vi "Get TableVariable Name List.vi"(8 "error in (no error)":errorcluster, 11 "DataTable":refnum<k7>) -> (0 "error out":errorcluster, 2 "TableVariable name list":string[](array[string]), 3 "DataTable out":refnum<k7>)   [LabVIEW 2019, in "JMP Automation.lvlib"]
doc: "retreive the name list of the TableVariable from a DataTable. The DataTable will be \"activated\" (put on the front) during the opperation\n\nDataTable: valide DataTable application handle"
uses:
  JMP Automation.lvlib
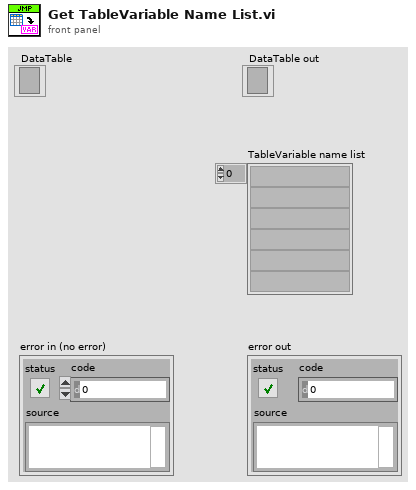
[diagram p1: front panel]
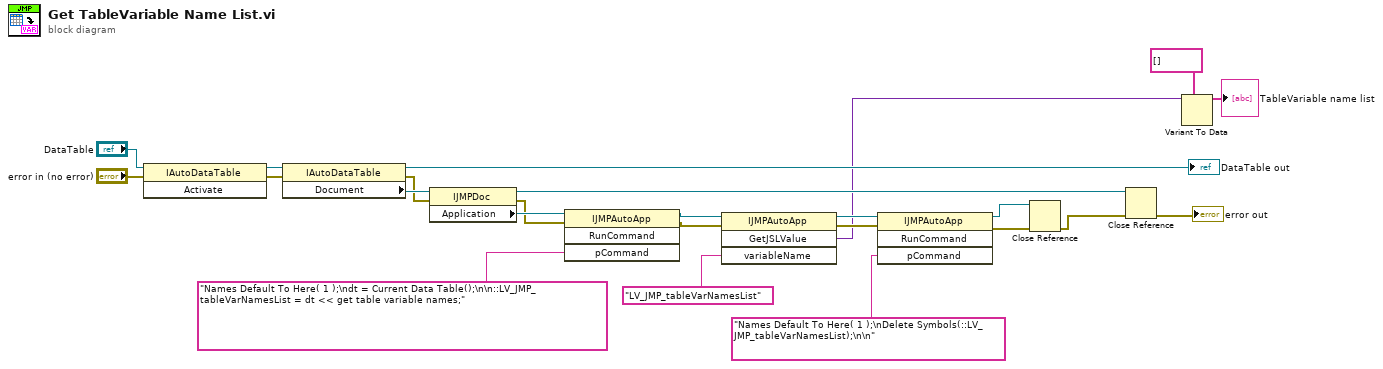
[diagram p0: block diagram]
diagram:
  n1 = invoke class="IAutoDataTable" method="Activate"(reference="DataTable", error in="error in (no error)") -> (reference out=w21:refnum<k7>, error out=w23:errorcluster)  [unwired: 1 in, 1 out]
  n2 = property class="IAutoDataTable"(reference=w21, error in=w23) -> (reference out=→"DataTable out":refnum<k7>, error out=w18:errorcluster, "Document"=w20:refnum<k7>)
  n3 = property class="IJMPDoc"(reference=w20, error in=w18) -> (reference out=w5:refnum<k7>, error out=w17:errorcluster, "Application"=w19:refnum<k7>)
  n4 = invoke class="IJMPAutoApp" method="RunCommand"(reference=w19, error in=w17, "pCommand"="Names Default To Here( 1 );\ndt = Current Data Table();\n\n::LV_JMP_tableVarNamesList = dt << get table variable names;") -> (reference out=w11:refnum<k7>, error out=w10:errorcluster)  [unwired: 1 in, 2 out]
  n5 = invoke class="IJMPAutoApp" method="GetJSLValue"(reference=w11, error in=w10, "variableName"="LV_JMP_tableVarNamesList") -> (reference out=w9:refnum<k7>, error out=w8:errorcluster, "GetJSLValue"=w1:variant)  [unwired: 1 in, 1 out]
  n6 = invoke class="IJMPAutoApp" method="RunCommand"(reference=w9, error in=w8, "pCommand"="Names Default To Here( 1 );\nDelete Symbols(::LV_JMP_tableVarNamesList);\n\n") -> (reference out=w7:refnum<k7>, error out=w6:errorcluster)  [unwired: 1 in, 2 out]
  n7 = Close Reference(reference=w7, error in (no error)=w6) -> (error out=w4:errorcluster)
  n8 = Close Reference(reference=w5, error in (no error)=w4) -> (error out=→"error out":errorcluster)
  n9 = Variant To Data(type=string[] [], Variant=w1) -> (data=→"TableVariable name list":string[])  [unwired: 1 in, 1 out]
